vi "remove from subscribers list.vi"(8 "error in (no error)":errorcluster, 10 "Subscriber Data":T1, 11 "RSeries_CAM in":refnum<class "RSeries_CAM.lvclass">) -> (0 "error out":errorcluster, 3 "RSeries_CAM out":refnum<class "RSeries_CAM.lvclass">)   [LabVIEW 2024, in "RSeries_CAM.lvlib" / "RSeries_CAM.lvclass"]
uses:
  RSeries_CAM.lvclass
  ARCH/Message Queue/Message Cluster.ctl
  RSeries_CAM.lvclass/RSeries_CAM.ctl
  ARCH/Message Queue/Message Queue.lvlib
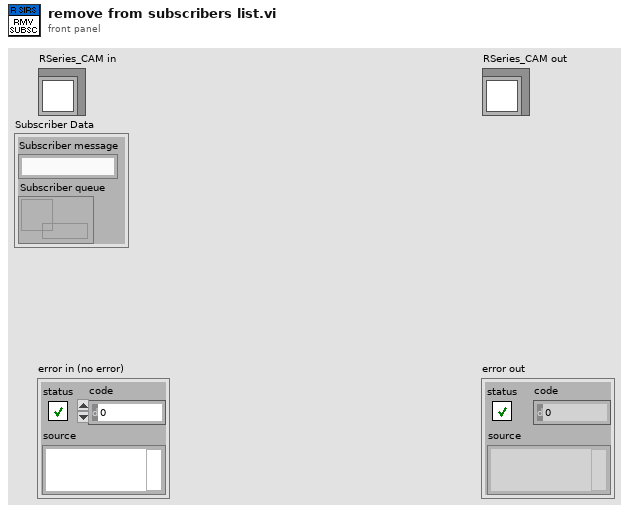
[diagram p1: front panel]
types:
  T1 = cluster{"Subscriber message":string, "Subscriber queue":refnum<queue>}
  T2 = cluster{"Subscriber message":string, "Subscriber queue":refnum<queue>}[]
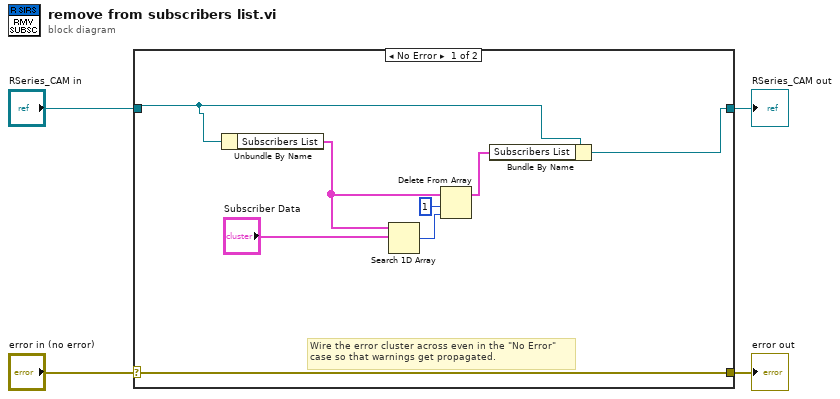
[diagram p0: block diagram]
diagram:
  n1 = case shown="No Error" "error in (no error)" {
    selector: "error in (no error)" -> [w12 w14]
    tunnel: [w12 w14] -> w3
    tunnel: [w10 w13] -> w1
    tunnel: "RSeries_CAM in" -> [w11 w13]
    frame No Error {
      # "Wire the error cluster across even in the \"No Error\"\ncase so that warnings get propagated."
      n2 = Unbundle By Name(w11) -> ("Subscribers List"=w8:T2)
      n3 = Search 1D Array(1D array=w8, element="Subscriber Data") -> (index of element=w7:i32)  [unwired: 1 in]
      n4 = Delete From Array(array=w8, length=1, index=w7) -> (array with subset deleted=w5:T2)  [unwired: 1 out]
      n5 = Bundle By Name(cluster=w11, "Subscribers List"=w5) -> (w10:refnum<class "RSeries_CAM.lvclass">)
    }
    frame Error {
    }
  }
  "error out" <- w3
  "RSeries_CAM out" <- w1
